vi "_PC_Spectrafilter calc_signal_of_noise_ratio.vi"(8 "error in (no error)":errorcluster, 9 "signal range":cluster{"start":dbl, "end":dbl}, 10 "noise feature":cluster{"noise diff":sgl, "median":dbl}, 11 "Spectrum in":cluster{"X":dbl[], "Y":sgl[]}) -> (0 "error out":errorcluster, 2 "ratio":dbl)   [LabVIEW 2018]
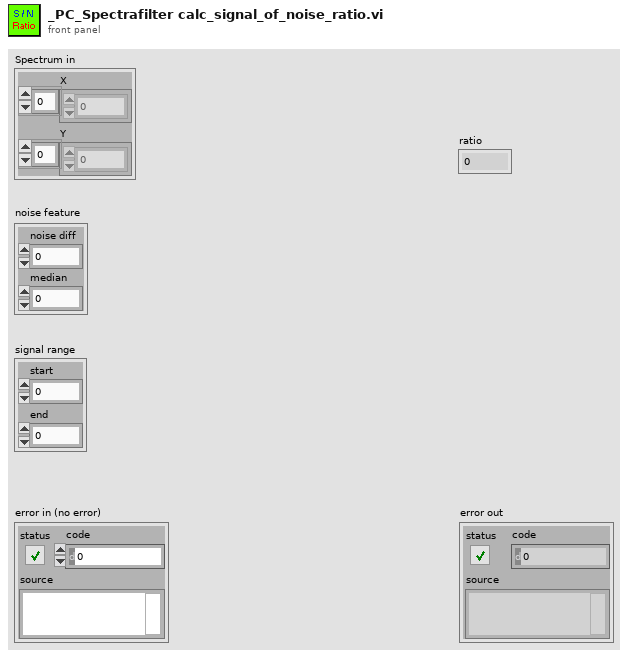
[diagram p1: front panel]
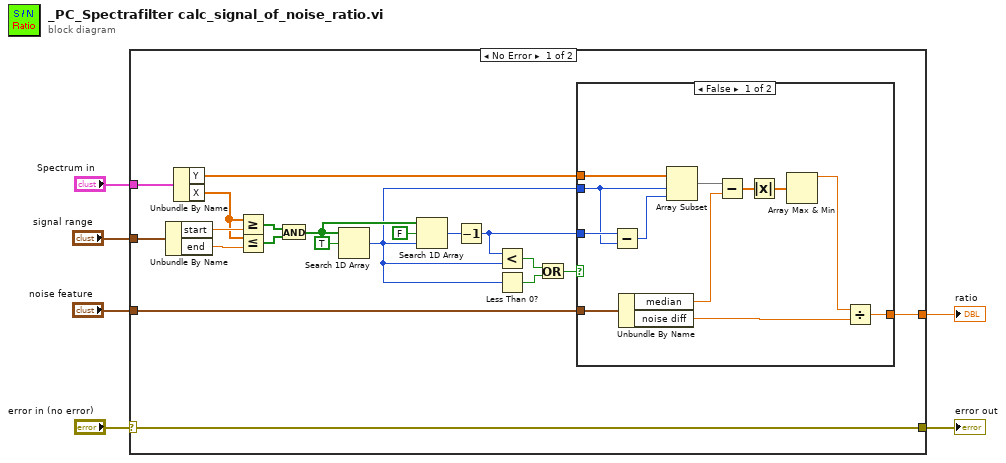
[diagram p0: block diagram]
diagram:
  n1 = case shown="No Error" "error in (no error)" {
    selector: "error in (no error)" -> [w26 _]
    tunnel: [w26 _] -> w5
    tunnel: "Spectrum in" -> [w14 _]
    tunnel: "signal range" -> [w17 _]
    tunnel: "noise feature" -> [w9 _]
    tunnel: [w7 _] -> w1
    frame No Error {
      n2 = Unbundle By Name(w17) -> ("start"=w16:dbl, "end"=w15:dbl)
      n3 = Unbundle By Name(w14) -> ("Y"=w8:sgl[], "X"=w13:dbl[])
      n4 = Greater Or Equal?(x=w13, y=w16) -> (x >= y?=w25:bool[])
      n5 = Less Or Equal?(x=w13, y=w15) -> (x <= y?=w24:bool[])
      n6 = And(x=w25, y=w24) -> (x .and. y?=w22:bool[])
      n7 = Search 1D Array(1D array=w22, element=TRUE) -> (index of element=w10:i32)  [unwired: 1 in]
      n8 = Search 1D Array(1D array=w22, element=FALSE, start index (0)=w10) -> (index of element=w20:i32)
      n9 = Decrement(x=w20) -> (x-1=w11:i32)
      n10 = Less?(x=w11, y=w10) -> (x < y?=w19:bool)
      n11 = Less Than 0?(x=w10) -> (x < 0?=w18:bool)
      n12 = Or(x=w19, y=w18) -> (x .or. y?=w12:bool)
      n13 = case shown="False" w12 {
        tunnel: w11 -> [w31 _]
        tunnel: w10 -> [w30 _]
        tunnel: w9 -> [w36 _]
        tunnel: w8 -> [w37 _]
        tunnel: [w32 _] -> w7
        frame False {
          n14 = Subtract(x=w31, y=w30) -> (x-y=w38:i32)
          n15 = Unbundle By Name(w36) -> ("median"=w35:dbl, "noise diff"=w33:sgl)
          n16 = Array Subset(array=w37, index=w30, length=w38) -> (w29:sgl[])
          n17 = Subtract(x=w29, y=w35) -> (x-y=w28:dbl[])
          n18 = Absolute Value(x=w28) -> (abs(x)=w27:dbl[])
          n19 = Array Max & Min(array=w27) -> (max value=w34:dbl)  [unwired: 3 out]
          n20 = Divide(x=w34, y=w33) -> (x/y=w32:dbl)
        }
        frame True {
        }
      }
    }
    frame Error {
    }
  }
  "error out" <- w5
  "ratio" <- w1
